vi "AddMassiveNombers (SubVI).vi"(11 "TblParam in":sgl[][](array[numeric])) -> (3 "TblParam out":sgl[][](array[numeric]))   [LabVIEW 2017]
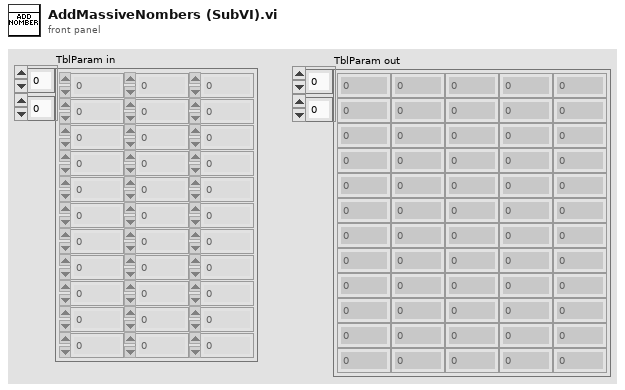
[diagram p1: front panel]
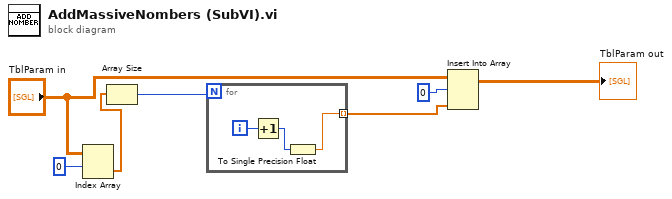
[diagram p0: block diagram]
diagram:
  n1 = Index Array(array="TblParam in", index (row)=0) -> (element=w2:sgl[])  [unwired: 1 in]
  n2 = Array Size(array=w2) -> (size(s)=w1:i32)
  n3 = for {
    N: w1 -> [_]
    tunnel: [w8] -> w6 mode=indexing
    i -> [w10]
    n4 = Increment(x=w10) -> (x+1=w9:i32)
    n5 = To Single Precision Float(number=w9) -> (single precision float=w8:sgl)
  }
  n6 = Insert Into Array(array="TblParam in", index (row)=0, new element=w6) -> (→"TblParam out":sgl[][])  [unwired: 1 in]
